vi "AcuiredDataRandom_SubVI.vi"() -> (3 "Array Out":u64[](array[numeric]))   [LabVIEW 2024]
uses:
  <vilib>/numeric/Random Number (Range) U64.vi
  <vilib>/numeric/sub_Random U32.vi
panel:
  out "error out":errorcluster
  in  "error in (no error)":errorcluster
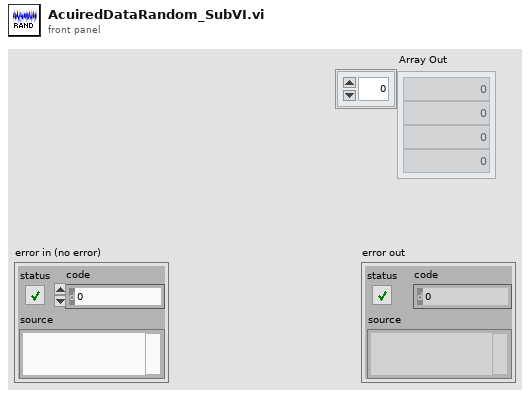
[diagram p1: front panel]
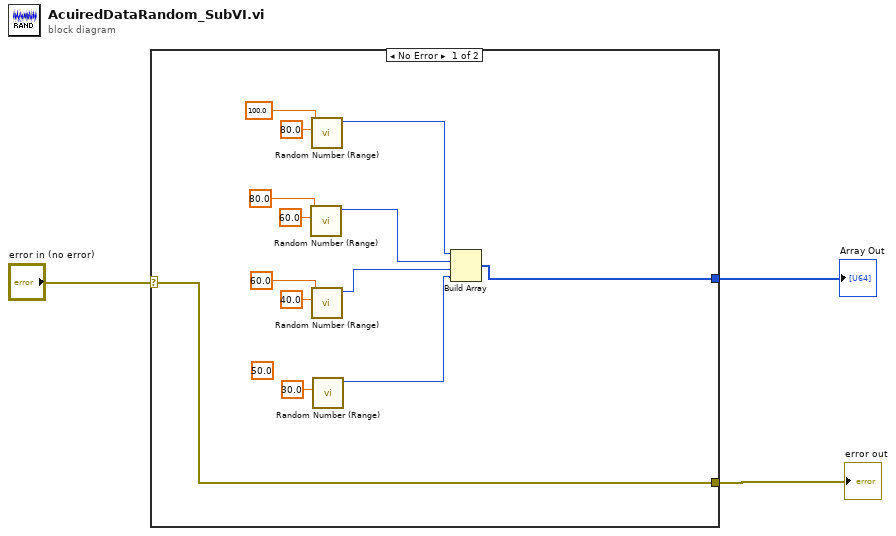
[diagram p0: block diagram]
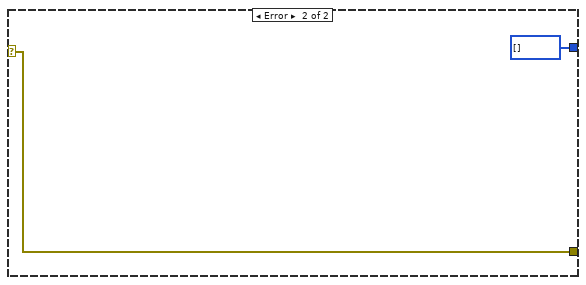
[diagram p2: hidden frame]
diagram:
  n1 = case shown="No Error" "error in (no error)" {
    selector: "error in (no error)" -> [w5 w18]
    tunnel: [w5 w18] -> w2
    tunnel: [w4 u64[] []] -> w1
    frame No Error {
      (unwired) 50.0 ("upper bound (100)")
      n2 = call-poly <vilib>:"Random Number (Range).vi"("lower bound (0)"=60.0, "upper bound (100)"=80.0) -> ("number"=w8:u64)  [unwired: 9 in]
      n3 = call-poly <vilib>:"Random Number (Range).vi"("lower bound (0)"=80.0, "upper bound (100)"=100.0) -> ("number"=w9:u64)  [unwired: 9 in]
      n4 = call-poly <vilib>:"Random Number (Range).vi"("lower bound (0)"=40.0, "upper bound (100)"=60.0) -> ("number"=w7:u64)  [unwired: 9 in]
      n5 = call-poly <vilib>:"Random Number (Range).vi"("lower bound (0)"=30.0) -> ("number"=w6:u64)  [unwired: 10 in]
      n6 = Build Array(w9, w8, w7, w6) -> (w4:u64[])
    }
    frame Error {
    }
  }
  "error out" <- w2
  "Array Out" <- w1
